vi "SendCommand.vi"(8 "error in":errorcluster, 10 "Command":string, 11 "T560Session in":refnum<class "T560Session.lvclass">) -> (0 "error out":errorcluster, 2 "Response":string, 3 "T560Session out":refnum<class "T560Session.lvclass">)   [LabVIEW 2013, in "T560Session.lvclass"]
uses:
  T560Session.lvclass
  T560Session.lvclass/T560Session.ctl
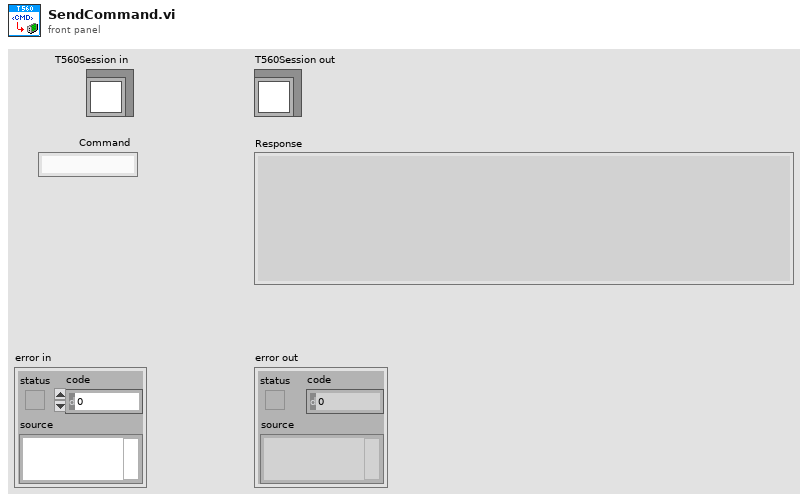
[diagram p1: front panel]
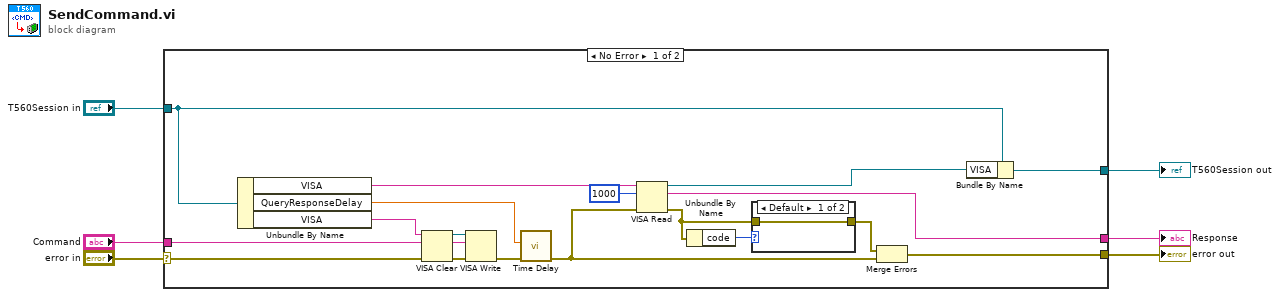
[diagram p0: block diagram]
diagram:
  n1 = case shown="No Error" "error in" {
    selector: "error in" -> [w7 w27]
    tunnel: [w11 w27] -> w5
    tunnel: [w24 w26] -> w3
    tunnel: "T560Session in" -> [w16 w26]
    tunnel: "Command" -> [w23 _]
    tunnel: [w20 _] -> w1
    frame No Error {
      n2 = Unbundle By Name(w16) -> ("VISA"=w18:string, "QueryResponseDelay"=w17:dbl, "VISA"=w8:string)
      n3 = VISA Clear(VISA resource name=w8, error in (no error)=w7) -> (VISA resource name out=w9:refnum<visa-resource-name>, error out=w10:errorcluster)
      n4 = VISA Write(VISA resource name=w9, write buffer=w23, error in (no error)=w10) -> (error out=w22:errorcluster)  [unwired: 2 out]
      n5 = call "Time Delay"("error in (no error)"=w22, "Delay Time (s)"=w17) -> ("error out"=w12:errorcluster)  [unwired: 9 in]
      n6 = VISA Read(VISA resource name=w18, byte count=u32 1000, error in (no error)=w12) -> (VISA resource name out=w21:refnum<visa-resource-name>, read buffer=w20:string, error out=w14:errorcluster)  [unwired: 1 out]
      n7 = Unbundle By Name(w14) -> ("code"=w15:i32)
      n8 = case shown="Default" w15 {
        tunnel: w14 -> [w25 _]
        tunnel: [w25 _] -> w13
        frame Default {
        }
        frame -1073807339 {
        }
      }
      n9 = Merge Errors(w13, w12) -> (w11:errorcluster)
      n10 = Bundle By Name(cluster=w16, "VISA"=w21) -> (w24:refnum<class "T560Session.lvclass">)
    }
    frame Error {
    }
  }
  "error out" <- w5
  "T560Session out" <- w3
  "Response" <- w1
